vi "MBtcp-OpenReadClose.vi"(4 "RegisterType":T1="Input", 5 "Slave ID":u8=255 format="%.0x", 6 "Timeout (900)":i32=900, 8 "error in (no error)":errorcluster, 9 "nRegisters":u16, 10 "RegisterAddr":u16, 11 "IP Address(:port)":string) -> (0 "error out":errorcluster, 1 "32bitValues":u32[](array[numeric]), 2 "16bitValues":u16[](array[numeric]))   [LabVIEW 2018]
uses:
  RegisterTypes.ctl
  <vilib>/Plasmionique/MB Master/MB_Master_TCP/MB_Master_TCP.lvclass
  Applications/National Instruments/LabVIEW 2018 64-bit/vi.lib/Plasmionique/MB Master/MB_Master/MB_Master.lvclass
  <vilib>/Plasmionique/MB Master/MB Master.lvlib
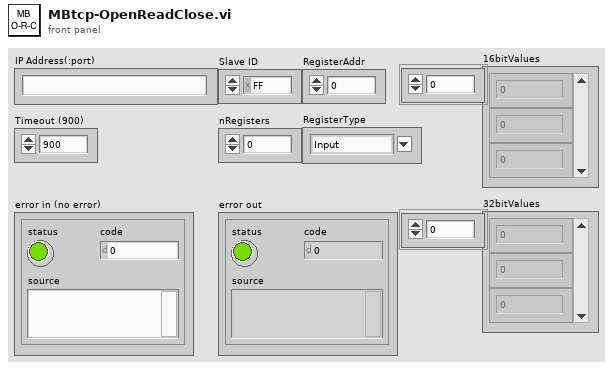
[diagram p1: front panel]
types:
  T1 = typedef "RegisterTypes.ctl" = string
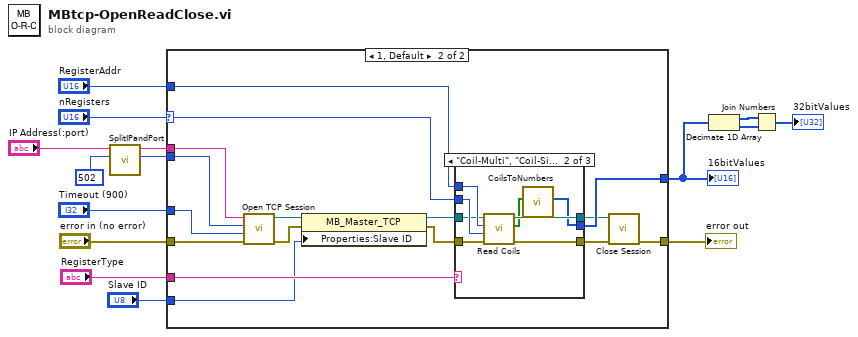
[diagram p0: block diagram]
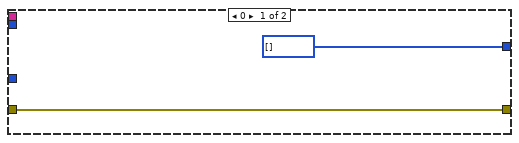
[diagram p2: hidden frame]
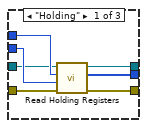
[diagram p3: hidden frame]
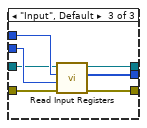
[diagram p4: hidden frame]
diagram:
  n1 = call "SplitIPandPort.vi"("defaultPort(10001)"=u16 502, "IP:Port"="IP Address(:port)") -> ("Port"=w1:u16, "IP"=w3:string)  [unwired: 8 in]
  n2 = case shown="1, Default" "nRegisters" {
    selector: "nRegisters" -> [_ w25]
    tunnel: [w17 w32] -> w15
    tunnel: [u16[] [] ("Registers") w31] -> w8
    tunnel: "RegisterAddr" -> [_ w30]
    tunnel: w3 -> [_ w29]
    tunnel: "error in (no error)" -> [w17 w28]
    tunnel: "Timeout (900)" -> [_ w27]
    tunnel: "RegisterType" -> [_ w20]
    tunnel: "Slave ID" -> [_ w19]
    tunnel: w1 -> [_ w18]
    frame 0 {
    }
    frame 1, Default {
      n3 = call <vilib>:"Open TCP Session.vi"("error in (no error)"=w28, "Timeout (10000)"=w27, "Port (502)"=w18, "IP Address"=w29) -> ("error out"=w22:errorcluster, "MB_TCP session"=w24:refnum<class "MB_Master_TCP.lvclass">)  [unwired: 6 in]
      n4 = property class="MB_Master_TCP"(reference=w24, error in=w22, "Properties:Slave ID"=w19) -> (reference out=w23:refnum<class "MB_Master_TCP.lvclass">, error out=w21:errorcluster)
      n5 = case shown="\"Coil-Multi\", \"Coil-Single\"" w20 {
        tunnel: [w40 w48 w55] -> w33
        tunnel: [w39 w41 w54] -> w31
        tunnel: w30 -> [w38 w47 w53]
        tunnel: [w37 w46 w52] -> w26
        tunnel: w25 -> [w36 w45 w51]
        tunnel: w23 -> [w35 w44 w50]
        tunnel: w21 -> [w34 w43 w49]
        frame "Holding" {
          n6 = call <vilib>:"Read Holding Registers.vi"("error in (no error)"=w34, "quantity"=w36, "starting address"=w38, "MB session in"=w35) -> ("error out"=w40:errorcluster, "Registers"=w39:u16[], "MB session out"=w37:refnum<class "MB_Master_TCP.lvclass">)  [unwired: 5 in]
        }
        frame "Coil-Multi", "Coil-Single" {
          n7 = call <vilib>:"Read Coils.vi"("error in (no error)"=w43, "quantity"=w45, "starting address"=w47, "MB session in"=w44) -> ("error out"=w48:errorcluster, "Coils"=w42:bool[], "MB session out"=w46:refnum<class "MB_Master_TCP.lvclass">)  [unwired: 5 in]
          n8 = call "CoilsToNumbers.vi"("Coils"=w42) -> ("16bitValues"=w41:u16[])  [unwired: 10 in]
        }
        frame "Input", Default {
          n9 = call <vilib>:"Read Input Registers.vi"("error in (no error)"=w49, "quantity"=w51, "starting address"=w53, "MB session in"=w50) -> ("error out"=w55:errorcluster, "Registers"=w54:u16[], "MB session out"=w52:refnum<class "MB_Master_TCP.lvclass">)  [unwired: 5 in]
        }
      }
      n10 = call-dynamic "Close Session.vi"("error in (no error)"=w33, "MB TCP session"=w26) -> ("error out"=w32:errorcluster)  [unwired: 9 in]
    }
  }
  "error out" <- w15
  "16bitValues" <- w8
  n11 = Decimate 1D Array(w8) -> (w9:u16[], w10:u16[])
  n12 = Join Numbers(hi=w9, lo=w10) -> ((hi.lo)=→"32bitValues":u32[])
